vi "file.vi"(7 "calling_vi":refnum<vi>, 8 "error in (no error)":errorcluster, 9 "filter":string="All files (*.*)|*.*", 10 "title":string, 11 "start_path":path) -> (0 "error out":errorcluster, 3 "selected_path":path)   [LabVIEW 2015, in "lv-dialog.lvlib"]
uses:
  System.Windows.Forms
  <vilib>/Utility/error.llb/Error Cluster From Error Code.vi
  <vilib>/ErrorRing/Error Ring.xnode
  lv-dialog.lvlib
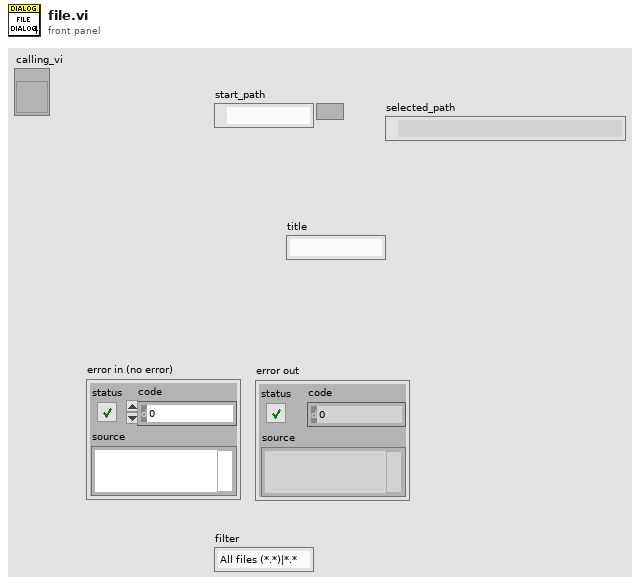
[diagram p1: front panel]
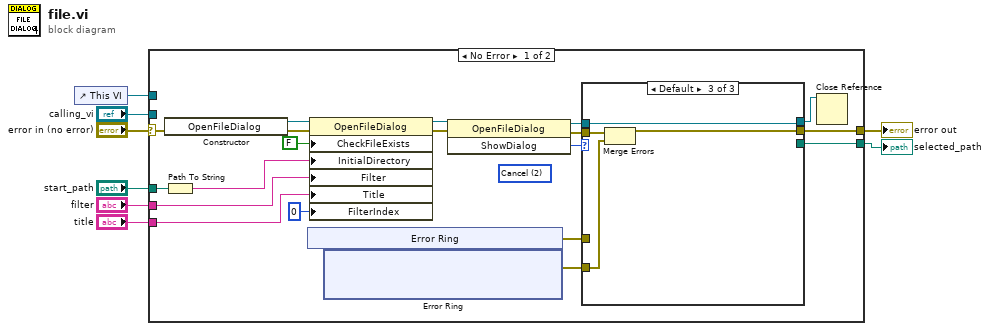
[diagram p0: block diagram]
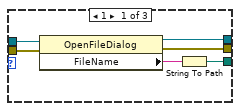
[diagram p2: hidden frame]
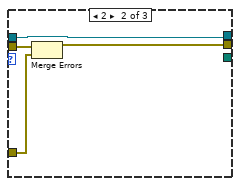
[diagram p3: hidden frame]
diagram:
  n1 = control-ref of="This VI"() -> (w5:refnum<vi>)
  n2 = case shown="No Error" "error in (no error)" {
    selector: "error in (no error)" -> [w27 w50]
    tunnel: [w23 w50] -> w7
    tunnel: "calling_vi" -> [_ _]
    tunnel: w5 -> [_ _]
    tunnel: "start_path" -> [w25 _]
    tunnel: "filter" -> [w26 _]
    tunnel: [w22 _] -> w2
    tunnel: "title" -> [w19 _]
    frame No Error {
      (unwired) 2 items=["None", "OK", "Cancel", "Abort", "Retry", "Ignore", "Yes", "No"] ("ShowDialog")
      n3 = constructor class="OpenFileDialog"(error in=w27) -> (reference out=w17:refnum<k24>, error out=w15:errorcluster)  [unwired: 2 in, 1 out]
      n4 = Path To String(path=w25) -> (string=w24:string)
      n5 = xnode "Error Ring"() -> ("error out"=w21:errorcluster)
      n6 = property class="OpenFileDialog"(reference=w17, error in=w15, "CheckFileExists"=FALSE, "InitialDirectory"=w24, "Filter"=w26, "Title"=w19, "FilterIndex"=0) -> (reference out=w16:refnum<k24>, error out=w14:errorcluster)
      n7 = xnode "Error Ring"() -> ("error out"=w20:errorcluster)
      n8 = invoke class="OpenFileDialog" method="ShowDialog"(reference=w16, error in=w14) -> (reference out=w13:refnum<k24>, error out=w12:errorcluster, "ShowDialog"=w11:i32)  [unwired: 1 in]
      n9 = case shown="Default" w11 {
        tunnel: w13 -> [w33 w34 w38]
        tunnel: w12 -> [w32 w37 w41]
        tunnel: [w29 _ _] -> w22
        tunnel: [w31 w36 w40] -> w23
        tunnel: w21 -> [_ w35 _]
        tunnel: w20 -> [_ _ w39]
        tunnel: [w28 w34 w38] -> w9
        frame 1 {
          n10 = property class="OpenFileDialog"(reference=w33, error in=w32) -> (reference out=w28:refnum<k24>, error out=w31:errorcluster, "FileName"=w30:string)
          n11 = String To Path(string=w30) -> (path=w29:path)
        }
        frame 2 {
          n12 = Merge Errors(w37, w35) -> (w36:errorcluster)
        }
        frame Default {
          n13 = Merge Errors(w41, w39) -> (w40:errorcluster)
        }
      }
      n14 = Close Reference(reference=w9) -> ()  [unwired: 1 in, 1 out]
    }
    frame Error {
    }
  }
  "error out" <- w7
  "selected_path" <- w2
